vi "Module Type.vi"(11 "SoftVar Module in":refnum<class "SoftVar Module.lvclass">) -> (2 "Module Type":string)   [LabVIEW 2020, in "Volatus.lvlib" / "SoftVar Module.lvclass"]
uses:
  SoftVar Module.lvclass
  SoftVar Module.lvclass/SoftVar Module.ctl
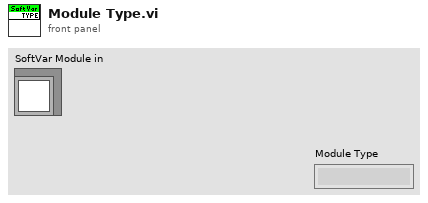
[diagram p1: front panel]
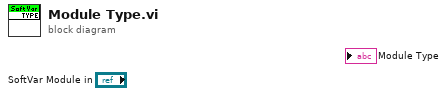
[diagram p0: block diagram]
diagram:
